vi "Open File.vi"(8 "error in (no error)":errorcluster, 10 "New File Path":path, 11 "File Writer in":refnum<class "File Writer.lvclass">) -> (0 "error out":errorcluster, 1 "Success?":bool, 3 "File Writer out":refnum<class "File Writer.lvclass">)   [LabVIEW 2020, in "File Writer.lvlib" / "File Writer.lvclass"]
doc: "Open a file by calling 'Open File Do'."
uses:
  File Writer.lvclass
  File Writer.lvclass/File Writer.ctl
  <vilib>/Utility/file.llb/Is Path and Not Empty.vi
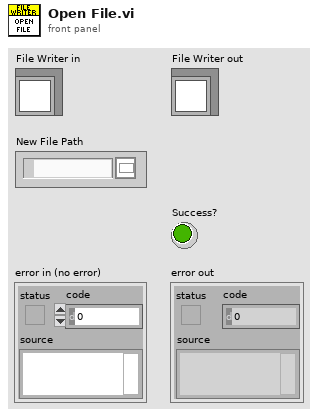
[diagram p1: front panel]
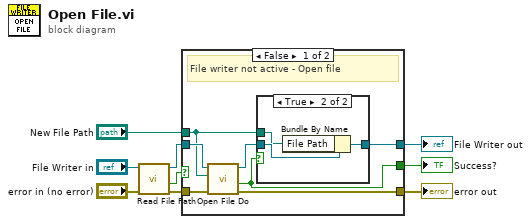
[diagram p0: block diagram]
diagram:
  n1 = call "Read File Path.vi"("error in (no error)"="error in (no error)", "File Writer in"="File Writer in") -> ("error out"=w2:errorcluster, "Is Active?"=w8:bool, "File Writer out"=w4:refnum<class "File Writer.lvclass">)  [unwired: 6 in, 1 out]
  n2 = case shown="False" w8 {
    tunnel: [w13 _] -> w7
    tunnel: "New File Path" -> [w10 _]
    tunnel: [w11 w22] -> w5
    tunnel: w4 -> [w16 w22]
    tunnel: w2 -> [w15 w21]
    tunnel: [w14 w21] -> w1
    frame False {
      # "File writer not active - Open file"
      n3 = call-dynamic "Open File Do.vi"("error in (no error)"=w15, "New File Path"=w10, "File Writer in"=w16) -> ("error out"=w14:errorcluster, "Success?"=w13:bool, "File Writer out"=w12:refnum<class "File Writer.lvclass">)  [unwired: 6 in]
      n4 = case shown="True" w13 {
        tunnel: [w17 w19] -> w11
        tunnel: w12 -> [w17 w20]
        tunnel: w10 -> [_ w18]
        frame False {
        }
        frame True {
          n5 = Bundle By Name(cluster=w20, "File Path"=w18) -> (w19:refnum<class "File Writer.lvclass">)
        }
      }
    }
    frame True {
      # "File writer active - Abort operation"
    }
  }
  "error out" <- w1
  "File Writer out" <- w5
  "Success?" <- w7
